vi "visa write read.vi"(6 "milliseconds to wait":u32=200, 8 "error in (no error)":errorcluster, 10 "write buffer":string="g", 11 "VISA resource name":refnum<visa-resource-name>="ASRL3::INSTR") -> (0 "error out":errorcluster={"status"=TRUE, "code"=-1073807346, "source"="VISA Clear in visa write read.vi"}, 2 "read buffer":string, 3 "VISA resource name out":refnum<visa-resource-name>)   [LabVIEW 2018]
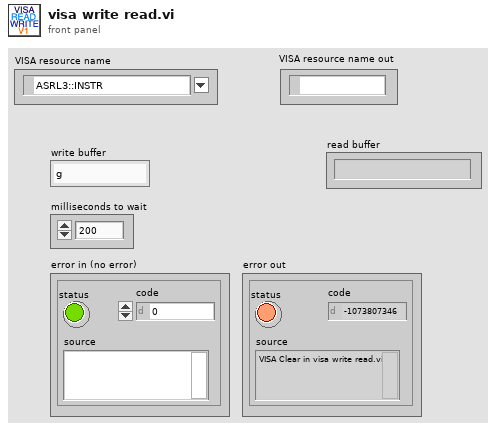
[diagram p1: front panel]
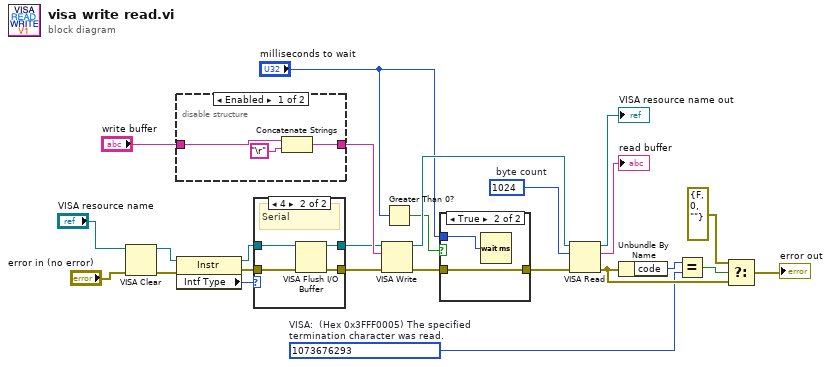
[diagram p0: block diagram]
diagram:
  w21 = 1073676293  # VISA:  (Hex 0x3FFF0005) The specified termination character was read.
  w18 = u32 1024  # byte count
  n1 = VISA Clear(VISA resource name="VISA resource name", error in (no error)="error in (no error)") -> (VISA resource name out=w3:refnum<visa-resource-name>, error out=w1:errorcluster)
  n2 = disable-structure shown="Enabled" {
    disable-tunnel: "write buffer" -> [w28 w29]
    disable-tunnel: [w27 w29] -> w14
    frame Enabled {
      n3 = Concatenate Strings(w28, "\r") -> (w27:string)
    }
    frame Disabled {
    }
  }
  n4 = property class="Instr"(reference=w3, error in=w1) -> (reference out=w8:refnum<visa-resource-name>, error out=w7:errorcluster, "Intf Type"=w9:u16)
  n5 = case shown="4" w9 {
    tunnel: w7 -> [w30 w35]
    tunnel: [w30 w34] -> w5
    tunnel: [w31 w33] -> w6
    tunnel: w8 -> [w31 w32]
    frame 0, Default {
    }
    frame 4 {
      # "Serial"
      n6 = VISA Flush I/O Buffer(VISA resource name=w32, error in (no error)=w35) -> (VISA resource name out=w33:refnum<visa-resource-name>, error out=w34:errorcluster)  [unwired: 1 in]
    }
  }
  n7 = VISA Write(VISA resource name=w6, write buffer=w14, error in (no error)=w5) -> (VISA resource name out=w17:refnum<visa-resource-name>, error out=w11:errorcluster)  [unwired: 1 out]
  n8 = Greater Than 0?(x="milliseconds to wait") -> (x > 0?=w13:bool)
  n9 = case shown="True" w13 {
    tunnel: "milliseconds to wait" -> [_ w38]
    tunnel: w11 -> [w36 w37]
    tunnel: [w36 w37] -> w10
    frame False {
    }
    frame True {
      n10 = Wait (ms)(milliseconds to wait=w38) -> ()  [unwired: 1 out]
    }
  }
  n11 = VISA Read(VISA resource name=w17, byte count=w18, error in (no error)=w10) -> (VISA resource name out=→"VISA resource name out":refnum<visa-resource-name>, read buffer=→"read buffer":string, error out=w23:errorcluster)  [unwired: 1 out]
  n12 = Unbundle By Name(w23) -> ("code"=w20:i32)
  n13 = Equal?(x=w20, y=w21) -> (x = y?=w24:bool)
  n14 = Select(t=errorcluster {"status"=FALSE, "code"=0, "source"=""}, s=w24, f=w23) -> (s? t:f=→"error out":errorcluster)
